vi "Vision Processing.vi"(4 "error in (no error)":errorcluster) -> ()   [LabVIEW 2018]
doc: "This VI runs in parallel to other tasks. It gets images from the camera, processes them for color or shape and uses commands or globals to affect the behavior of other subsystems."
uses:
  <vilib>/Rock Robotics/WPI/Camera/WPI_CameraImageSize.ctl
  <vilib>/Rock Robotics/WPI/Camera/WPI_CameraExposure Values.ctl
  <vilib>/Rock Robotics/WPI/Camera/WPI_CameraWhite Balance Values.ctl
  <vilib>/Rock Robotics/WPI/Camera/WPI_CameraFrameRate.ctl
  Framework/Robot Global Data.vi
  <vilib>/Rock Robotics/Network Tables/NT Write Number.vi
  <vilib>/Rock Robotics/Network Tables/NT Read Boolean.vi
  <vilib>/Rock Robotics/Network Tables/NT Write Boolean.vi
panel:
  in  "error in (no error) 2":errorcluster
  in  "Image Size":T1=enum."320x240"
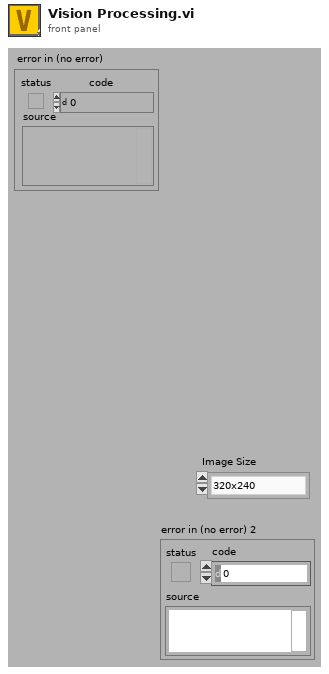
[diagram p1: front panel]
types:
  T1 = typedef "WPI_CameraImageSize.ctl" = enum16{"640x480", "320x240", "160x120", "Custom"}
  T2 = typedef "WPI_CameraFrameRate.ctl" = u32
  T3 = typedef "WPI_CameraExposure Values.ctl" = enum16{"Auto", "Flicker-free 50 Hz", "Flicker-free 60 Hz", "Hold current", "Custom"}
  T4 = typedef "WPI_CameraWhite Balance Values.ctl" = enum16{"Auto", "Fixed indoor", "Fixed outdoor 1", "Fixed outdoor 2", "Fixed fluorescent 1", "Fixed fluorescent 2", "Hold current", "Custom"}
  T5 = typedef "Image Type" = u32
  T6 = typedef "WPI_CameraDevRef.ctl" = cluster{"Camera Address":string, "CameraStatus":errorcluster}
  T7 = typedef "IMAQ Image.ctl" = refnum<image>
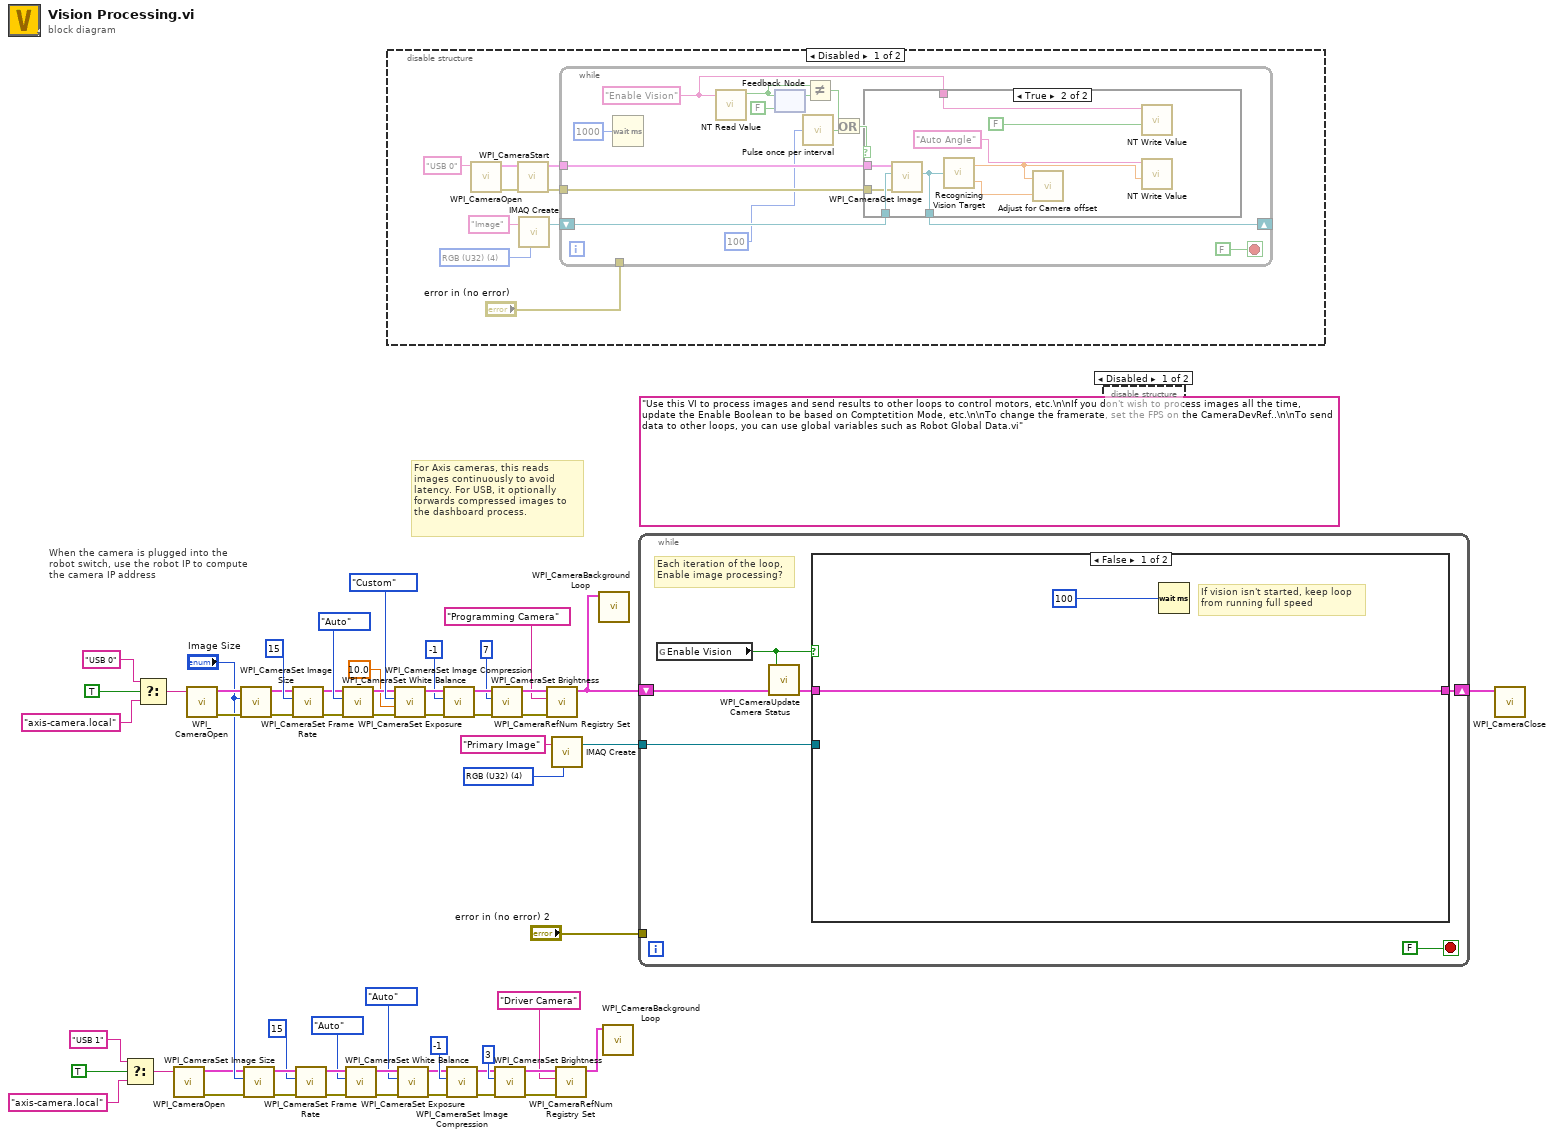
[diagram p0: block diagram]
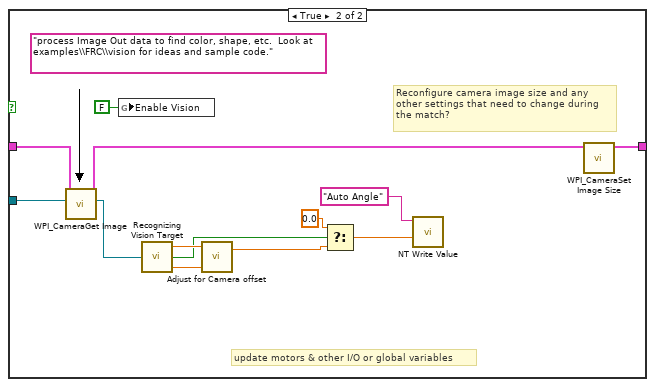
[diagram p4: hidden frame]
diagram:
  (unwired) "Use this VI to process images and send results to other loops to control motors, etc.\n\nIf you don't wish to process images all the time, update the Enable Boolean to be based on Comptetition Mode, etc.\n\nTo change the framerate, set the FPS on the CameraDevRef..\n\nTo send data to other loops, you can use global variables such as Robot Global Data.vi"
  w28 = T5 4 items=["Grayscale (U8)", "Grayscale (I16)", "Grayscale (SGL)", "Complex (CSG)", "RGB (U32)", "HSL (U32)", "RGB (U64)"] ("Image Type")
  # "When the camera is plugged into the\nrobot switch, use the robot IP to compute\nthe camera IP address"
  # "For Axis cameras, this reads\nimages continuously to avoid\nlatency. For USB, it optionally\nforwards compressed images to\nthe dashboard process."
  n1 = Select(t="USB 1" ("format string"), s=TRUE ("dot notation? (F)"), f="axis-camera.local" ("format string")) -> (s? t:f=w6:string)
  n2 = Select(t="USB 0" ("format string"), s=TRUE ("dot notation? (F)"), f="axis-camera.local" ("format string")) -> (s? t:f=w56:string)
  n3 = call <vilib>:"WPI_CameraOpen.vi"("Camera Address"=w6) -> ("error out"=w17:errorcluster, "CameraDevRef"=w18:T6)  [unwired: 1 in, 8 out]
  n4 = call <vilib>:"WPI_CameraOpen.vi"("Camera Address"=w56) -> ("error out"=w40:errorcluster, "CameraDevRef"=w39:T6)  [unwired: 1 in, 8 out]
  n5 = call <vilib>:"WPI_CameraSet Image Size.vi"("error in (no error)"=w40, "Image Size"="Image Size", "CameraDevRef"=w39) -> ("error out"=w41:errorcluster, "CameraDevRef Out"=w38:T6)  [unwired: 1 in, 6 out]
  n6 = call <vilib>:"WPI_CameraSet Image Size.vi"("error in (no error)"=w17, "Image Size"="Image Size", "CameraDevRef"=w18) -> ("error out"=w16:errorcluster, "CameraDevRef Out"=w19:T6)  [unwired: 1 in, 6 out]
  n7 = call <vilib>:"WPI_CameraSet Frame Rate.vi"("error in (no error)"=w41, "Frame Rate (fps)"=T2 15, "CameraDevRef"=w38) -> ("error out"=w42:errorcluster, "CameraDevRef Out"=w36:T6)  [unwired: 7 out]
  n8 = call <vilib>:"WPI_CameraSet Frame Rate.vi"("error in (no error)"=w16, "Frame Rate (fps)"=T2 15, "CameraDevRef"=w19) -> ("error out"=w15:errorcluster, "CameraDevRef Out"=w21:T6)  [unwired: 7 out]
  n9 = call <vilib>:"WPI_CameraSet White Balance.vi"("error in (no error)"=w42, "White Balance"=WPI_CameraWhite_Balance_Values."Auto", "CameraDevRef"=w36) -> ("error out"=w43:errorcluster, "CameraDevRef Out"=w37:T6)  [unwired: 1 in, 6 out]
  n10 = call <vilib>:"WPI_CameraSet White Balance.vi"("error in (no error)"=w15, "White Balance"=WPI_CameraWhite_Balance_Values."Auto", "CameraDevRef"=w21) -> ("error out"=w14:errorcluster, "CameraDevRef Out"=w20:T6)  [unwired: 1 in, 6 out]
  n11 = disable-structure shown="Disabled" {
    frame Disabled {
      w58 = T5 4 items=["Grayscale (U8)", "Grayscale (I16)", "Grayscale (SGL)", "Complex (CSG)", "RGB (U32)", "HSL (U32)", "RGB (U64)", "Grayscale (U16)"] ("Image Type")
      n12 = call <vilib>:"WPI_CameraOpen.vi"("Camera Address"="USB 0") -> ("error out"=w61:errorcluster, "CameraDevRef"=w62:T6)  [unwired: 9 in]
      n13 = call <vilib>:"WPI_CameraStart.vi"("error in (no error)"=w61, "CameraDevRef"=w62) -> ("error out"=w65:errorcluster, "CameraDevRef"=w64:T6)  [unwired: 8 in]
      n14 = call "IMAQ Create"("Image Name"="Image", "Image Type"=w58) -> ("New Image"=w63:T7)  [unwired: 3 in, 1 out]
      n15 = while {
        shift-right: [w79] -> _
        shift-left: w63 -> [w80]
        tunnel: w64 -> [w78]
        tunnel: w65 -> [w77]
        tunnel: "error in (no error)" -> [_]
        stop <- FALSE stop-if-true
        w73 = "Enable Vision" ("Name")
        n16 = Wait (ms)(milliseconds to wait=u32 1000) -> ()  [unwired: 1 out]
        n17 = call-poly <vilib>:"NT Read Value.vi"("Name"=w73) -> ("Boolean"=w76:bool)  [unwired: 9 in, 1 out]
        n18 = feedback-in #1(w76) -> ()
        n19 = feedback #1(FALSE ("Boolean")) -> (w75:bool)
        n20 = call "Pulse once per interval.vi"("Time (ms)"=u32 100 ("milliseconds to wait")) -> ("Boolean"=w70:bool)
        n21 = Not Equal?(x=w76, y=w75) -> (x != y?=w71:bool)
        n22 = Or(x=w71, y=w70) -> (x .or. y?=w69:bool)
        n23 = case shown="True" w69 {
          tunnel: w80 -> [w81 w90]
          tunnel: [w81 w84] -> w79
          tunnel: w78 -> [_ w89]
          tunnel: w77 -> [_ w88]
          tunnel: w73 -> [_ w87]
          frame False {
          }
          frame True {
            n24 = call <vilib>:"WPI_CameraGet Image.vi"("error in (no error)"=w88, "Image"=w90, "CameraDevRef"=w89) -> ("Image Out"=w84:T7)  [unwired: 6 in, 2 out]
            n25 = call "Recognizing Vision Target.vi"("Image Src"=w84) -> ("Angle 2"=w83:dbl, "Distance (ft)"=w82:dbl)
            n26 = call "Adjust for Camera offset.vi"("Distance"=w82, "Angle"=w83) -> ()  [unwired: 2 out]
            n27 = call-poly <vilib>:"NT Write Value.vi"("Boolean"=FALSE, "Name"=w87) -> ()  [unwired: 9 in, 1 out]
            n28 = call-poly <vilib>:"NT Write Value.vi"("Numeric"=w83, "Name"="Auto Angle") -> ()  [unwired: 9 in, 1 out]
          }
        }
      }
    }
    frame Enabled {
    }
  }
  n29 = call <vilib>:"WPI_CameraSet Exposure.vi"("error in (no error)"=w43, "Exposure (%)"=10.0, "Exposure"=WPI_CameraExposure_Values."Custom", "CameraDevRef"=w37) -> ("error out"=w44:errorcluster, "CameraDevRef Out"=w34:T6)  [unwired: 6 out]
  n30 = call <vilib>:"WPI_CameraSet Exposure.vi"("error in (no error)"=w14, "Exposure"=WPI_CameraExposure_Values."Auto", "CameraDevRef"=w20) -> ("error out"=w13:errorcluster, "CameraDevRef Out"=w23:T6)  [unwired: 1 in, 6 out]
  n31 = call <vilib>:"WPI_CameraSet Image Compression.vi"("error in (no error)"=w44, "Compression"=-1, "CameraDevRef"=w34) -> ("error out"=w45:errorcluster, "CameraDevRef Out"=w35:T6)  [unwired: 7 out]
  n32 = call <vilib>:"WPI_CameraSet Image Compression.vi"("error in (no error)"=w13, "Compression"=-1, "CameraDevRef"=w23) -> ("error out"=w12:errorcluster, "CameraDevRef Out"=w22:T6)  [unwired: 7 out]
  n33 = call <vilib>:"WPI_CameraSet Brightness.vi"("error in (no error)"=w45, "Brightness"=7, "CameraDevRef"=w35) -> ("error out"=w47:errorcluster, "CameraDevRef Out"=w46:T6)  [unwired: 1 in, 6 out]
  n34 = call <vilib>:"WPI_CameraSet Brightness.vi"("error in (no error)"=w12, "Brightness"=3, "CameraDevRef"=w22) -> ("error out"=w3:errorcluster, "CameraDevRef Out"=w4:T6)  [unwired: 1 in, 6 out]
  n35 = call <vilib>:"WPI_CameraRefNum Registry Set.vi"("error in (no error)"=w47, "refnum name"="Programming Camera", "CameraDevRef"=w46) -> ("CameraDevRef"=w51:T6)  [unwired: 1 in, 7 out]
  n36 = call "IMAQ Create"("Image Name"="Primary Image", "Image Type"=w28) -> ("New Image"=w30:T7)  [unwired: 2 in, 2 out]
  n37 = call <vilib>:"WPI_CameraRefNum Registry Set.vi"("error in (no error)"=w3, "refnum name"="Driver Camera", "CameraDevRef"=w4) -> ("CameraDevRef"=w1:T6)  [unwired: 1 in, 7 out]
  n38 = call <vilib>:"WPI_CameraBackground Loop.vi"("CameraDevRef"=w51) -> ()  [unwired: 11 in]
  n39 = call <vilib>:"WPI_CameraBackground Loop.vi"("CameraDevRef"=w1) -> ()  [unwired: 11 in]
  n40 = while {
    shift-right: [w95] -> w52
    shift-left: w51 -> [w93]
    tunnel: w30 -> [w94]
    tunnel: "error in (no error) 2" -> [_]
    stop <- FALSE stop-if-true
    # "Each iteration of the loop,\nEnable image processing?"
    n41 = global read "Robot Global Data.vi" "Enable Vision"() -> (w91:bool)
    n42 = call <vilib>:"WPI_CameraUpdate Camera Status.vi"("CameraDevRef In"=w93, "Enable Vision"=w91) -> ("CameraDevRef Out"=w92:T6)  [unwired: 3 in]
    n43 = case shown="False" w91 {
      tunnel: w94 -> [_ w110]
      tunnel: [w98 w111] -> w95
      tunnel: w92 -> [w98 w109]
      frame False {
        # "If vision isn't started, keep loop\nfrom running full speed"
        n44 = Wait (ms)(milliseconds to wait=u32 100) -> ()  [unwired: 1 out]
      }
      frame True {
        (unwired) "process Image Out data to find color, shape, etc.  Look at examples\\FRC\\vision for ideas and sample code."
        # "update motors & other I/O or global variables"
        # "Reconfigure camera image size and any\nother settings that need to change during\nthe match?"
        n45 = call <vilib>:"WPI_CameraGet Image.vi"("Image"=w110, "CameraDevRef"=w109) -> ("Image Out"=w105:T7, "CameraDevRef Out"=w108:T6)  [unwired: 1 in, 7 out]
        n46 = global write "Robot Global Data.vi" "Enable Vision"(FALSE ("Enable Vision")) -> ()
        n47 = call "Recognizing Vision Target.vi"("Image Src"=w105) -> ("Distance (ft)"=w101:dbl, "Boolean"=w103:bool, "Angle 2"=w107:dbl)  [unwired: 2 in]
        n48 = call "Adjust for Camera offset.vi"("Distance"=w101, "Angle"=w107) -> ("Angle"=w100:dbl)  [unwired: 1 out]
        n49 = Select(t=0.0, s=w103, f=w100) -> (s? t:f=w102:dbl)
        n50 = call-poly <vilib>:"NT Write Value.vi"("Numeric"=w102, "Name"="Auto Angle") -> ()  [unwired: 9 in, 1 out]
        n51 = call <vilib>:"WPI_CameraSet Image Size.vi"("CameraDevRef"=w108) -> ("CameraDevRef Out"=w111:T6)  [unwired: 3 in, 7 out]
      }
    }
  }
  n52 = disable-structure shown="Disabled" {
    frame Disabled {
    }
    frame Enabled {
    }
  }
  n53 = call <vilib>:"WPI_CameraClose.vi"("CameraDevRef"=w52) -> ()  [unwired: 1 in, 10 out]
